vi "Initialise String Texture.vi"(6 "Wrap Length [pixels]":i32, 8 "error in (no error)":errorcluster, 9 "Name":string, 10 "Text":string, 11 "Font Combo":string) -> (0 "error out":errorcluster, 3 "Name In Cache":string)   [LabVIEW 2015, in "Resource Manager.lvclass"]
uses:
  Resource Manager.lvclass
  Texture/Texture.lvclass/Texture.ctl
  Resource Manager.lvclass/Resource Manager.ctl
  LabSDL2/Source/Libraries/LibSDL2 Wrapper/Destroy Texture.vi
  Globals.vi
  Texture/Texture.lvclass
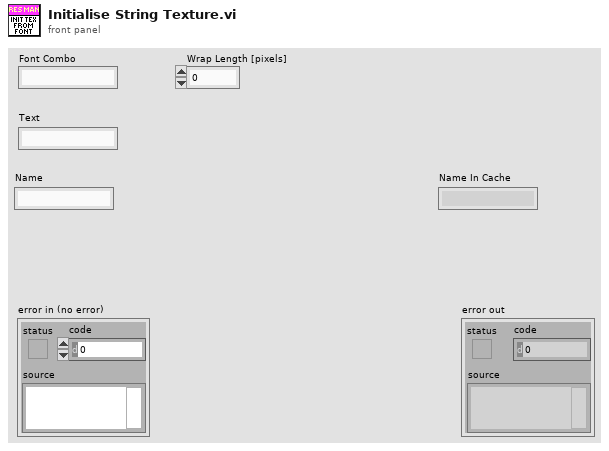
[diagram p1: front panel]
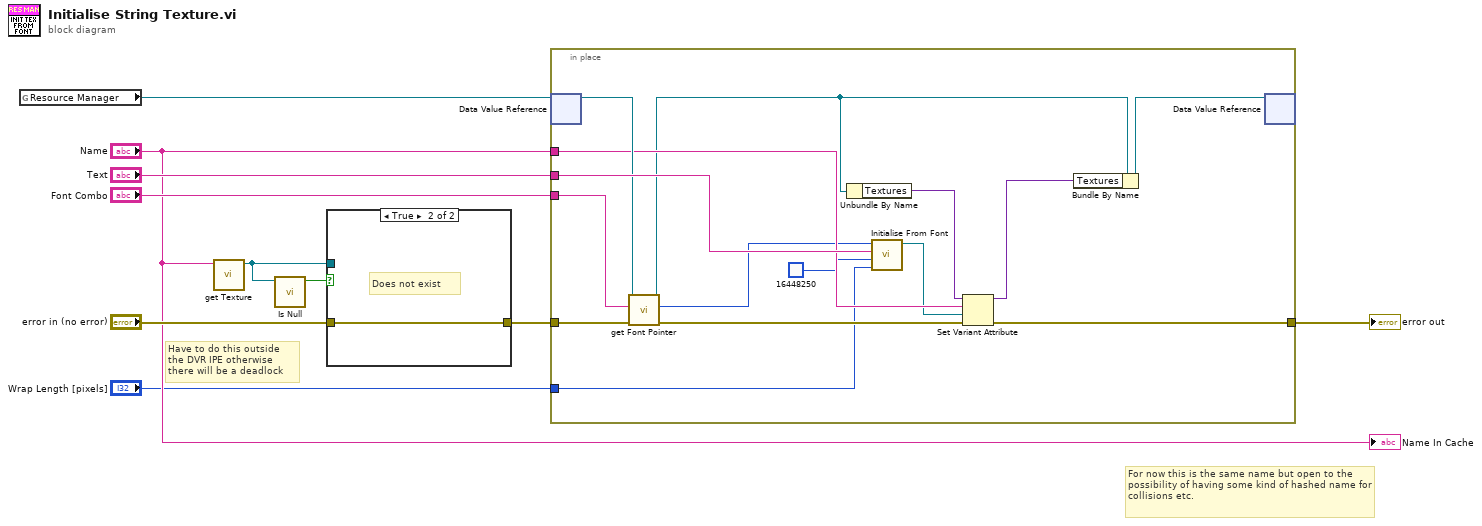
[diagram p0: block diagram]
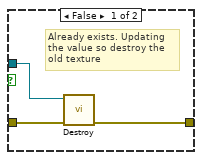
[diagram p2: hidden frame]
diagram:
  # "Have to do this outside the DVR IPE otherwise there will be a deadlock"
  # "For now this is the same name but open to the possibility of having some kind of hashed name for collisions etc."
  n1 = global read "Globals.vi" "Resource Manager"() -> (w7:refnum<data-value>)
  n2 = call "get Texture.vi"("Texture Name"="Name") -> ("Texture"=w6:refnum<class "Texture.lvclass">)  [unwired: 10 in]
  n3 = call "Is Null.vi"("Texture in"=w6) -> ("Is Null"=w5:bool)  [unwired: 10 in]
  n4 = case shown="True" w5 {
    tunnel: "error in (no error)" -> [w13 w14]
    tunnel: [w12 w14] -> w3
    tunnel: w6 -> [w11 _]
    frame False {
      # "Already exists. Updating the value so destroy the old texture"
      n5 = call "Destroy.vi"("error in (no error)"=w13, "Texture in"=w11) -> ("error out"=w12:errorcluster)  [unwired: 9 in]
    }
    frame True {
      # "Does not exist"
    }
  }
  n6 = in-place {
    in-place-border: [w29] -> w10
    in-place-border: "Name" -> [w25]
    in-place-border: "Text" -> [w27]
    in-place-border: "Font Combo" -> [w24]
    in-place-border: w3 -> [w17]
    in-place-border: "Wrap Length [pixels]" -> [w15]
    n7 = in-place-dvr #1(w7) -> (w26:refnum<class "Resource Manager.lvclass">)  [unwired: 1 out]
    n8 = call "get Font Pointer.vi"("error in (no error)"=w17, "Font Combo"=w24, "Resource Manager in"=w26) -> ("error out"=w20:errorcluster, "Font Pointer"=w18:u32, "Resource Manager out"=w19:refnum<class "Resource Manager.lvclass">)  [unwired: 6 in]
    n9 = Unbundle By Name(w19) -> ("Textures"=w23:variant)
    n10 = call "Initialise From Font.vi"("Wrap Length [pixels]"=w15, "Colour"=u32 16448250, "Text"=w27, "Font Pointer"=w18) -> ("Texture out"=w21:refnum<class "Texture.lvclass">)  [unwired: 7 in]
    n11 = Set Variant Attribute(Variant=w23, name=w25, value=w21, error in=w20) -> (Variant out=w22:variant, error out=w29:errorcluster)  [unwired: 1 out]
    n12 = Bundle By Name(cluster=w19, "Textures"=w22) -> (w28:refnum<class "Resource Manager.lvclass">)
    n13 = in-place-dvr #1(w28) -> ()  [unwired: 2 out]
  }
  "error out" <- w10
  "Name In Cache" <- "Name"
